vi "jobbatchColumn.vi"() -> ()   [LabVIEW 2012]
uses:
  <vilib>/addons/database/Auxilliary.llb/DB Tools DataTypes.ctl
  <vilib>/addons/database/Connection.llb/DB Tools Open Connec (Path).vi
  <vilib>/addons/database/NI_Database_API.lvlib
panel:
  out "column information":T2(array[cluster])
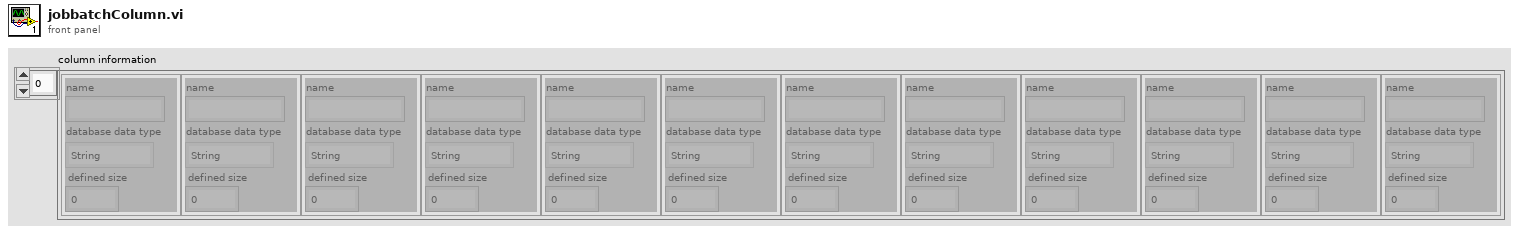
[diagram p1: front panel]
types:
  T1 = typedef "NI_Database_API.lvlib/DB Tools DataTypes.ctl" = enum16{"String", "Long (I32)", "Single (SGL)", "Double (DBL)", "Date/Time", "Binary"}
  T2 = cluster{"name":string, "database data type":T1, "defined size":i32}[]
  T3 = typedef "NI_Database_API.lvlib/Conn ObjectReference.ctl" = refnum<k1>
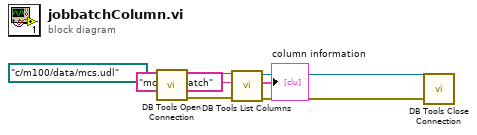
[diagram p0: block diagram]
diagram:
  n1 = call-poly <vilib>:"DB Tools Open Connection.vi"("connection information"=path "c:/m100/data/mcs.udl") -> ("error out"=w6:errorcluster, "connection reference"=w7:T3)  [unwired: 7 in]
  n2 = call <vilib>:"DB Tools List Columns.vi"("error in (no error)"=w6, "table"="mcs_jobbatch", "connection reference"=w7) -> ("error out"=w4:errorcluster, "column information"=→"column information":T2, "connection reference out"=w5:T3)  [unwired: 1 in, 1 out]
  n3 = call <vilib>:"DB Tools Close Connection.vi"("error in (no error)"=w4, "connection reference"=w5) -> ()  [unwired: 5 in, 1 out]
